vi "Concatenate Arrays.vi"(8 "error in (no error)":errorcluster, 9 "JSON Datatypes":refnum<class "JSON Value.lvclass">[](array[class]), 11 "JSON Array in":refnum<class "JSON Value.lvclass">) -> (0 "error out":errorcluster, 2 "JSON Array out":refnum<class "JSON Value.lvclass">)   [LabVIEW 2017, in "JSON Value.lvclass"]
doc: "Adds multiple elements to the end of a JSON Array"
uses:
  JSON Value.lvclass
  JSON Value.lvclass/JSON Value.ctl
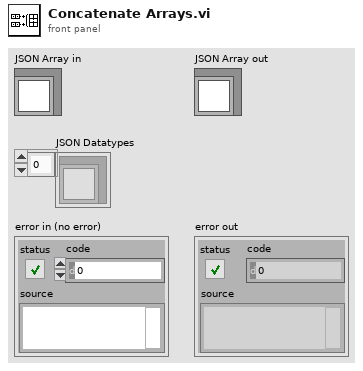
[diagram p1: front panel]
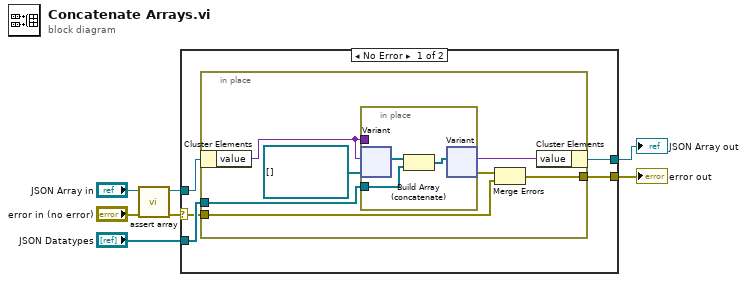
[diagram p0: block diagram]
diagram:
  n1 = call "assert array.vi"("error in (no error)"="error in (no error)", "JSON Value in"="JSON Array in") -> ("error out"=w4:errorcluster, "JSON Value out"=w2:refnum<class "JSON Value.lvclass">)  [unwired: 8 in]
  n2 = case shown="No Error" w4 {
    selector: w4 -> [w9 w23]
    tunnel: w2 -> [w12 w24]
    tunnel: [w11 w24] -> w7
    tunnel: "JSON Datatypes" -> [w10 _]
    tunnel: [w8 w23] -> w1
    frame No Error {
      n3 = in-place {
        in-place-border: w10 -> [w19]
        in-place-border: w9 -> [w14]
        in-place-border: [w13] -> w8
        n4 = in-place-cluster #1(w12) -> ("value"=w17:variant)
        n5 = in-place {
          in-place-border: w19 -> [w22]
          in-place-border: w17 -> [_]
          n6 = in-place-variant #2(w17, refnum<class "JSON Value.lvclass">[] [] ("JSON Datatypes")) -> (w21:refnum<class "JSON Value.lvclass">[])  [unwired: 1 out]
          n7 = Build Array (concatenate)(w21, w22) -> (w20:refnum<class "JSON Value.lvclass">[])
          n8 = in-place-variant #2(w20) -> (w16:variant, w15:errorcluster)
        }
        n9 = Merge Errors(w15, w14) -> (w13:errorcluster)
        n10 = in-place-cluster #1("value"=w16) -> (w11:refnum<class "JSON Value.lvclass">)
      }
    }
    frame Error {
    }
  }
  "JSON Array out" <- w7
  "error out" <- w1
